vi "sensor cmd write flash block.vi"(7 "length":u32, 9 "data":string, 10 "address":u32, 11 "device_handle":u32) -> (1 "data out":string, 2 "function return":i32, 3 "device_handle out":u32)   [LabVIEW 2019, in "apdm.lvlib"]
doc: "APDM_EXPORT int apdm_sensor_cmd_write_flash_block(apdm_device_handle_t device_handle, const uint32_t address, uint8_t *data, const uint32_t length);"
uses:
  apdm.lvlib
  Lee Lab/CP FES Walking 2018/Code/Working/LabVIEW/apdm.dll
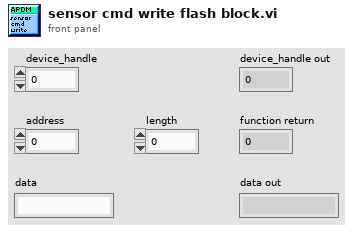
[diagram p1: front panel]
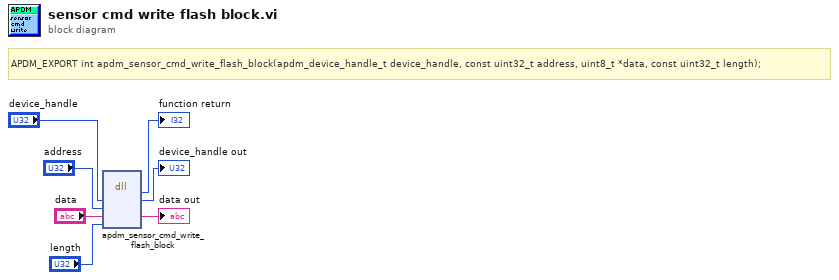
[diagram p0: block diagram]
diagram:
  # "APDM_EXPORT int apdm_sensor_cmd_write_flash_block(apdm_device_handle_t device_handle, const uint32_t address, uint8_t *data, const uint32_t length);"
  n1 = dll-call lib="C:/Users/jfalesi/Dropbox/Lee Lab/CP FES Walking 2018/Code/Working/LabVIEW/apdm.*" fn="apdm_sensor_cmd_write_flash_block"("device_handle"="device_handle", "address"="address", "data"="data", "length"="length") -> (→"function return":i32, "device_handle"=→"device_handle out":u32, "data"=→"data out":string)  [unwired: 5 in, 2 out]
